vi "Get FPGA Dependent File.vi"(8 "error in (no error)":errorcluster, 11 "ID in":T1 format="%.0x") -> (0 "error out":errorcluster, 1 "Windows Path":path, 2 "RT Path":path, 3 "ID out":T1 format="%.0x")   [LabVIEW 2011, in "Engine Sim System Explorer.lvlib"]
uses:
  <vilib>/NI Veristand/Custom Device API/Custom Device Item Ref.ctl
  NationalInstruments.VeriStand.SystemDefinitionAPI
  Engine Sim System Explorer.lvlib
  <vilib>/NI Veristand/Custom Device Offline API/Custom Device Offline API.lvlib
  <vilib>/NI Veristand/Custom Device API/Custom Device API.lvlib
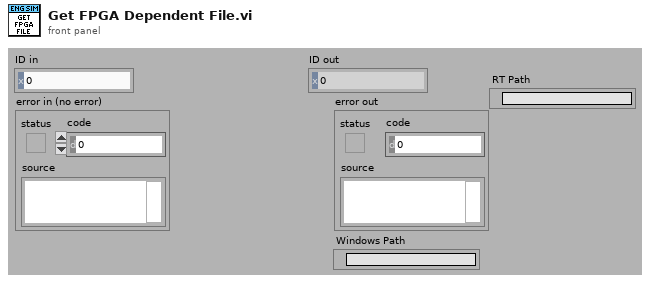
[diagram p1: front panel]
types:
  T1 = typedef "Custom Device API.lvlib/Custom Device Item Ref.ctl" = u64
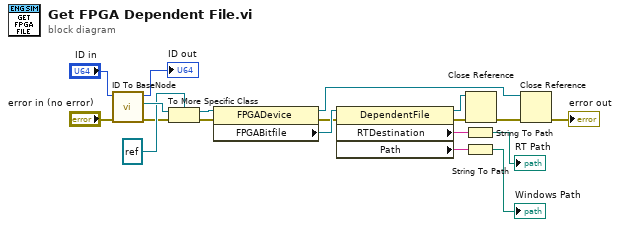
[diagram p0: block diagram]
diagram:
  n1 = call <vilib>:"ID To BaseNode.vi"("error in (no error)"="error in (no error)", "ID in"="ID in") -> ("error out"=w17:errorcluster, "BaseNode"=w19:refnum<k24>, "ID out"=→"ID out":u64)  [unwired: 7 in]
  n2 = To More Specific Class(target class=refnum<k24> refnum ("BaseNodeType"), reference=w19, error in=w17) -> (specific class reference=w16:refnum<k24>, error out=w15:errorcluster)
  n3 = property class="FPGADevice"(reference=w16, error in=w15) -> (reference out=w10:refnum<k24>, error out=w8:errorcluster, "FPGABitfile"=w9:refnum<k24>)
  n4 = property class="DependentFile"(reference=w9, error in=w8) -> (reference out=w6:refnum<k24>, error out=w7:errorcluster, "RTDestination"=w4:string, "Path"=w2:string)
  n5 = String To Path(string=w4) -> (path=→"RT Path":path)
  n6 = String To Path(string=w2) -> (path=→"Windows Path":path)
  n7 = Close Reference(reference=w6, error in (no error)=w7) -> (error out=w5:errorcluster)
  n8 = Close Reference(reference=w10, error in (no error)=w5) -> (error out=→"error out":errorcluster)
